vi "AO Wait Until Done.vi"(8 "error in (no error)":errorcluster, 10 "Params":variant, 11 "NI Analog Output in":refnum<class "NI Analog Output.lvclass">) -> (0 "error out":errorcluster, 3 "NI Analog Output out":refnum<class "NI Analog Output.lvclass">)   [LabVIEW 2020, in "NI DAQmx.lvlib" / "NI Analog Output.lvclass"]
uses:
  NI Analog Output.lvclass
  D:/WSGitHub/RTFWK/Realization/NI DAQmx Base/NI DAQmx Base.lvclass
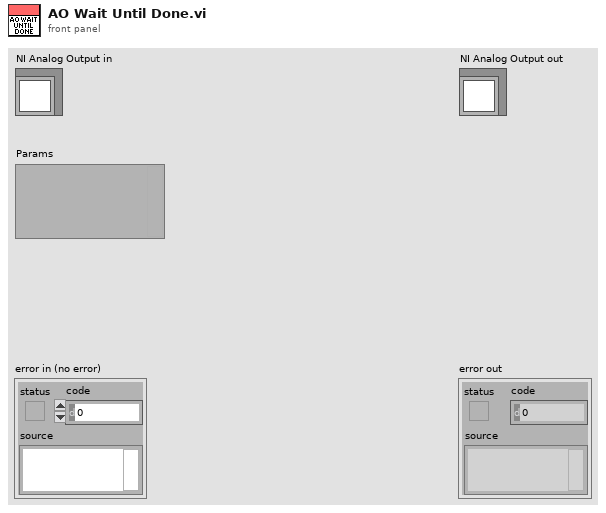
[diagram p1: front panel]
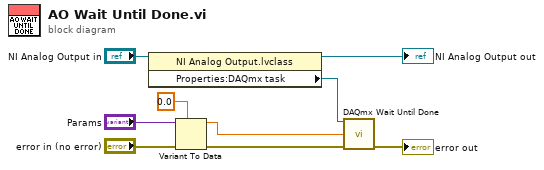
[diagram p0: block diagram]
diagram:
  n1 = property class="NI Analog Output.lvclass"(reference="NI Analog Output in") -> (reference out=→"NI Analog Output out":refnum<class "NI Analog Output.lvclass">, "Properties:DAQmx task"=w4:refnum<k21>)  [unwired: 1 in, 1 out]
  n2 = Variant To Data(error in="error in (no error)", type=0.0, Variant="Params") -> (data=w1:dbl, error out=w5:errorcluster)
  n3 = call <vilib>:"DAQmx Wait Until Done.vi"("task/channels in"=w4, "timeout (sec)"=w1, "error in"=w5) -> ("error out"=→"error out":errorcluster)  [unwired: 11 in, 1 out]
